vi "Init.vi"(7 "Prepend Result Name":bool, 8 "error in (no error)":errorcluster, 9 "SA Pin":string, 10 "Measurement Name":string) -> (0 "error out":errorcluster, 3 "SpecAn_CHP out":refnum<class "SpecAn_CHP.lvclass">)   [LabVIEW 2018, in "SeqAuto Evaluations.lvlib" / "SpecAn_CHP.lvclass"]
uses:
  SpecAn_CHP.lvclass
  C:/Sequence Automation/Plugins/SeqAuto IEvaluation.lvlibp/SeqAuto IEvaluation.lvclass
  SpecAn_CHP.lvclass/SpecAn_CHP.ctl
  Write SA Pin.vi
  Plugins/SeqAuto IEvaluation.lvlibp/Write Measurement Name.vi
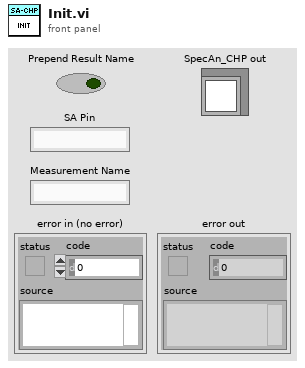
[diagram p1: front panel]
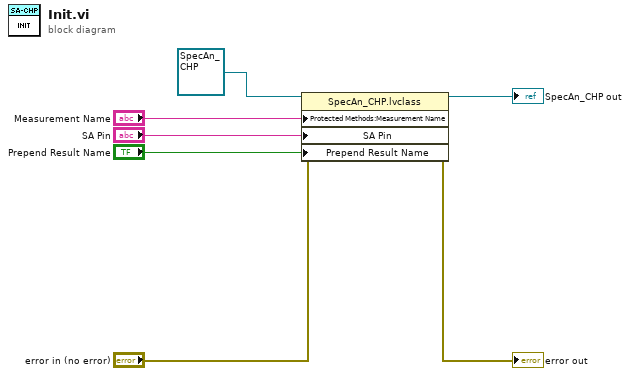
[diagram p0: block diagram]
diagram:
  n1 = property class="SpecAn_CHP.lvclass"(reference=refnum<class "SpecAn_CHP.lvclass"> refnum ("SpecAn_CHP in"), error in="error in (no error)", "Protected Methods:Measurement Name"="Measurement Name", "SA Pin"="SA Pin", "Prepend Result Name"="Prepend Result Name") -> (reference out=→"SpecAn_CHP out":refnum<class "SpecAn_CHP.lvclass">, error out=→"error out":errorcluster)
